vi "UI.vi"() -> ()   [LabVIEW 2013]
panel:
  out "PCB temp":dbl[](array[slide]) scale=0.0..200.0
  in  "PCB config":u16(ring)
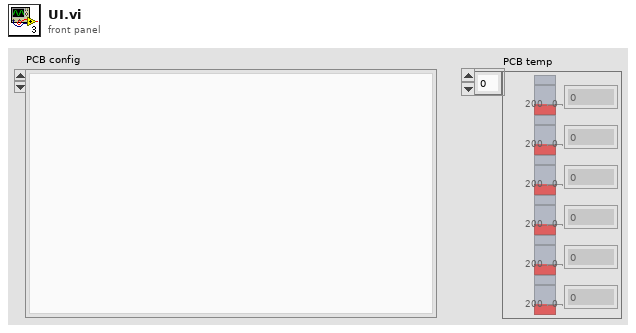
[diagram p1: front panel]
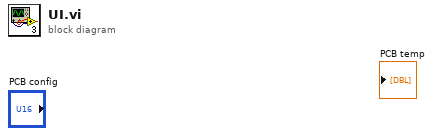
[diagram p0: block diagram]
diagram:
